vi "RandomColor.vi"(11 "Index":i32=-1) -> (3 "Color":u32(colorbox))   [LabVIEW 2020, in "LcPictureBox.lvclass"]
doc: "Generate colors that are good for a white background and distinguishable from each other.\n\nAuthored by David A. Moore\nsupport@mooregoodideas.com\nwww.mooregoodideas.com\n\nCopyright (c) 2010, Moore Good Ideas, Inc.\n\nAll rights reserved.\n\nRedistribution and use in source and binary forms, with or without modification, are permitted provided that the following conditions are met:\n\n * Redistributions of source code must retain the above copyright notice, this list of conditions and the following disclaimer.\n * Redistributions in binary form must reproduce the above copyright notice, this list of conditions and the following disclaimer in the documentation and/or other materials provided with the distribution.\n * Neither the name of Moore Good Ideas, Inc. nor the names of its contributors may be used to endorse or promote products derived from this software without specific prior written permission.\n\nTHIS SOFTWARE IS PROVIDED BY THE COPYRIGHT HOLDERS AND CONTRIBUTORS \"AS IS\" AND ANY EXPRESS OR IMPLIED WARRANTIES, INCLUDING, BUT NOT LIMITED TO, THE IMPLIED WARRANTIES OF MERCHANTABILITY AND FITNESS FOR A PARTICULAR PURPOSE ARE DISCLAIMED. IN NO EVENT SHALL THE COPYRIGHT OWNER OR CONTRIBUTORS BE LIABLE FOR ANY DIRECT, INDIRECT, INCIDENTAL, SPECIAL, EXEMPLARY, OR CONSEQUENTIAL DAMAGES (INCLUDING, BUT NOT LIMITED TO, PROCUREMENT OF SUBSTITUTE GOODS OR SERVICES; LOSS OF USE, DATA, OR PROFITS; OR BUSINESS INTERRUPTION) HOWEVER CAUSED AND ON ANY THEORY OF LIABILITY, WHETHER IN CONTRACT, STRICT LIABILITY, OR TORT (INCLUDING NEGLIGENCE OR OTHERWISE) ARISING IN ANY WAY OUT OF THE USE OF THIS SOFTWARE, EVEN IF ADVISED OF THE POSSIBILITY OF SUCH DAMAGE."
uses:
  LcPictureBox.lvclass
  <vilib>/numeric/Random Number (Range) U64.vi
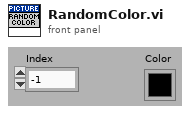
[diagram p1: front panel]
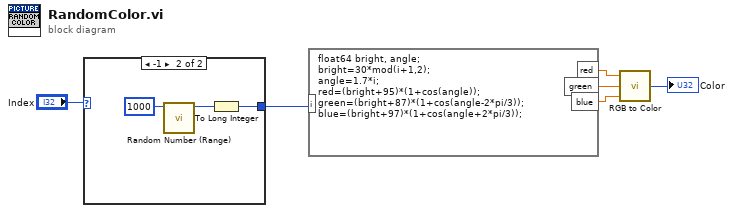
[diagram p0: block diagram]
diagram:
  n1 = case shown="-1" "Index" {
    selector: "Index" -> [w7 _]
    tunnel: [w7 w8] -> w1
    frame 0, Default {
    }
    frame -1 {
      n2 = call-poly <vilib>:"Random Number (Range).vi"("upper bound (100)"=u64 1000) -> ("number"=w9:u64)  [unwired: 10 in]
      n3 = To Long Integer(number=w9) -> (32bit integer=w8:i32)
    }
  }
  n4 = formula code="float64 bright, angle;\nbright=30*mod(i+1,2);\nangle=1.7*i;\nred=(bright+95)*(1+cos(angle));\ngreen=(bright+87)*(1+cos(angle-2*pi/3));\nblue=(bright+97)*(1+cos(angle+2*pi/3));"("i"=w1) -> ("red"=w5:dbl, "green"=w6:dbl, "blue"=w4:dbl)
  n5 = call <vilib>:"RGB to Color.vi"("B"=w4, "G"=w6, "R"=w5) -> ("Color"=→"Color":u32)
